vi "StateMachineTimer.vi"(11 "When to rollover":i32=1500) -> (3 "Current  Time in ms":i32)   [LabVIEW 2014]
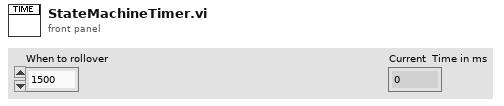
[diagram p1: front panel]
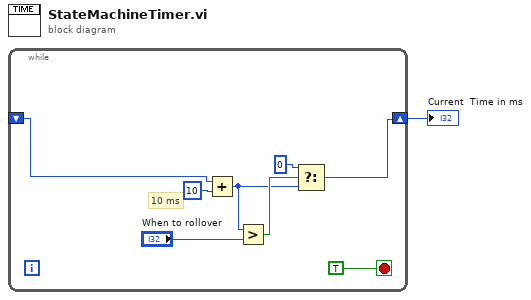
[diagram p0: block diagram]
diagram:
  n1 = while {
    shift-right: [w3] -> w1
    shift-left: _ -> [w2]
    stop <- TRUE stop-if-true
    # "10 ms"
    n2 = Add(x=w2, y=10) -> (x+y=w4:i32)
    n3 = Greater?(x=w4, y="When to rollover") -> (0:w6:bool)
    n4 = Select(t=0, s=w6, f=w4) -> (s? t:f=w3:i32)
  }
  "Current  Time in ms" <- w1
